vi "Main.vi"(8 "error in":errorcluster, 11 "UART Worker in":refnum<class "UART Worker.lvclass">) -> (0 "error out":errorcluster, 3 "UART Worker out":refnum<class "UART Worker.lvclass">)   [LabVIEW 2020, in "UART Worker.lvclass"]
doc: "The <b>Queued Message Handler</b> of the Worker that owns this VI."
uses:
  UART Worker.lvclass
  C:/Program Files (x86)/National Instruments/LabVIEW 2020/vi.lib/addons/_Workers/Library/Classes/Worker/Worker.lvclass
  rqp_Open Port.ctl
  rqp_Write Buffer.ctl
  Initialization Data.ctl
  Response Cases.ctl
  UART Worker.lvclass/UART Worker.ctl
  rql_readBuffer.ctl
  rql_checkBufferSize.ctl
  rql_checkBufferData.ctl
  rqp_Close Port.ctl
  <vilib>/Utility/error.llb/Error Cluster From Error Code.vi
  <vilib>/ErrorRing/Error Ring.xnode
  <vilib>/addons/_Workers/Library/Classes/Message Queue/Message Queue.lvclass
  3fd13485-57e7-4225-91d7-578f471f1d53.vi
panel:
  in  "stop":bool
  in  "讀取目標字數":i32=1
  in  "Write":bool
  in  "VISA resource name":refnum<visa-resource-name>
  out "read buffer":string
  in  "write buffer":string
  # "1. 設定 VISA\n2. 設定讀取目標字數\n3. 按下”開始通訊”，進行通訊作業\n4. 設定\"write buffer“\n5. 按下\"Write\"，將資料進行寫入\n6. 觀察\"read buffer\"\n7. 按下停止通訊“，結束通訊作業"
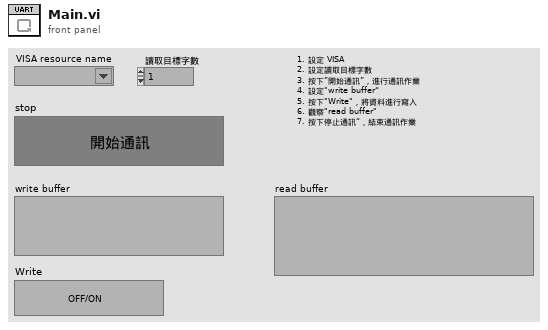
[diagram p1: front panel]
types:
  T1 = typedef "UART Worker.lvclass/Initialization Data.ctl" = cluster{"Response Cases":T2}
  T2 = typedef "UART Worker.lvclass/Response Cases.ctl" = cluster{"Placeholder - Can be deleted":string}
  T3 = typedef "UART Worker.lvclass/rql_checkBufferSize.ctl" = cluster{"Buffer Data":string}
  T4 = typedef "UART Worker.lvclass/rql_readBuffer.ctl" = cluster{"Number of Bytes at Serial Port":u32}
  T5 = typedef "UART Worker.lvclass/rql_checkBufferData.ctl" = cluster{"String":string}
  T6 = typedef "UART Worker.lvclass/rqp_Open Port.ctl" = cluster{"VISA resource name":refnum<visa-resource-name>}
  T7 = typedef "UART Worker.lvclass/rqp_Close Port.ctl" = cluster{"String":string}
  T8 = typedef "UART Worker.lvclass/rqp_Write Buffer.ctl" = cluster{"write buffer":string}
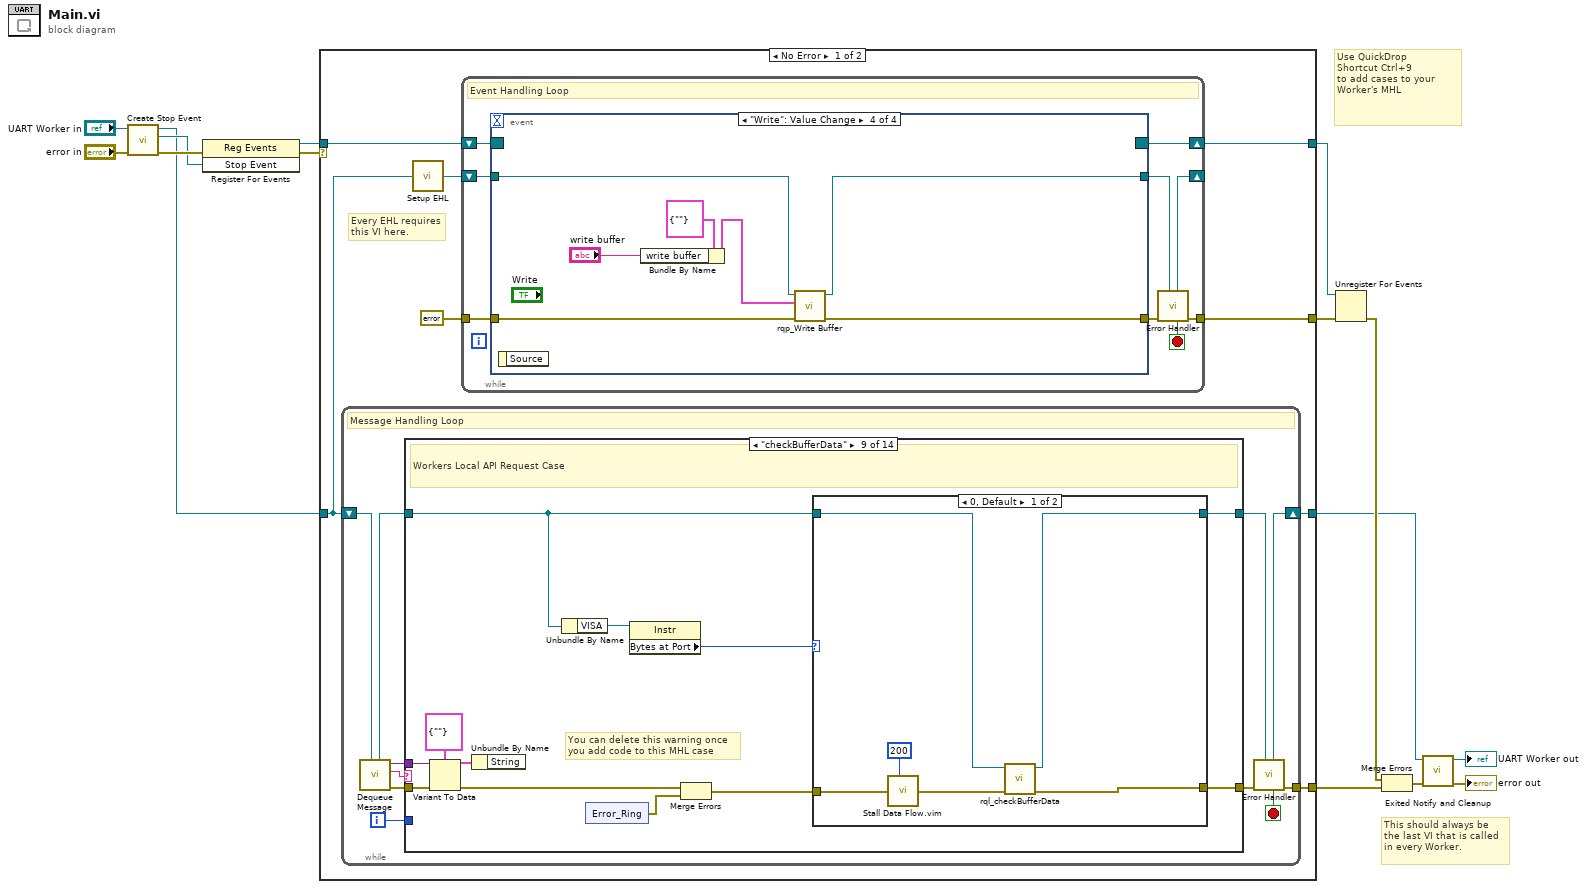
[diagram p0: block diagram]
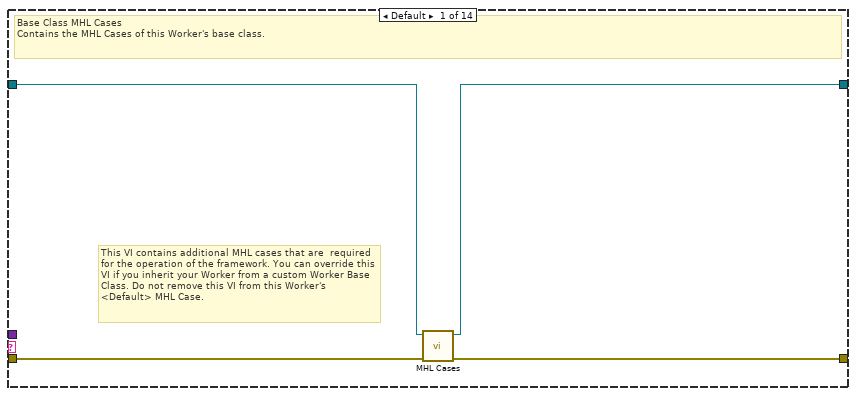
[diagram p2: hidden frame]
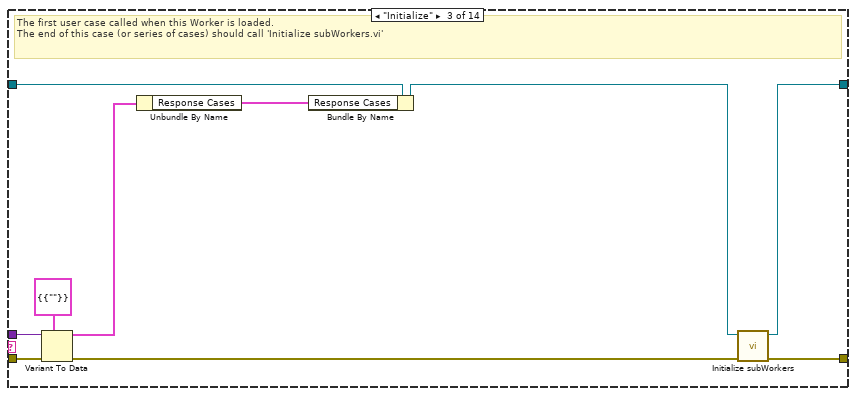
[diagram p4: hidden frame]
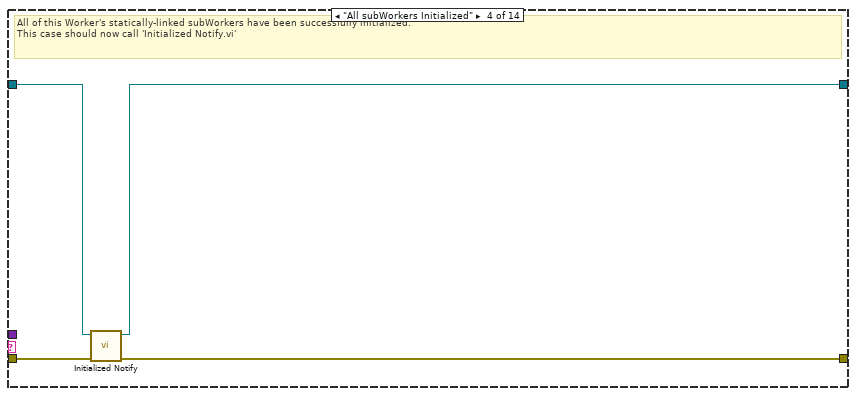
[diagram p5: hidden frame]
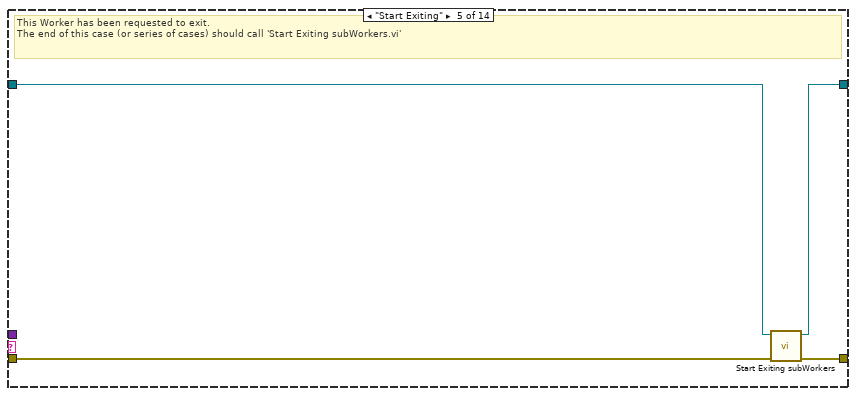
[diagram p6: hidden frame]
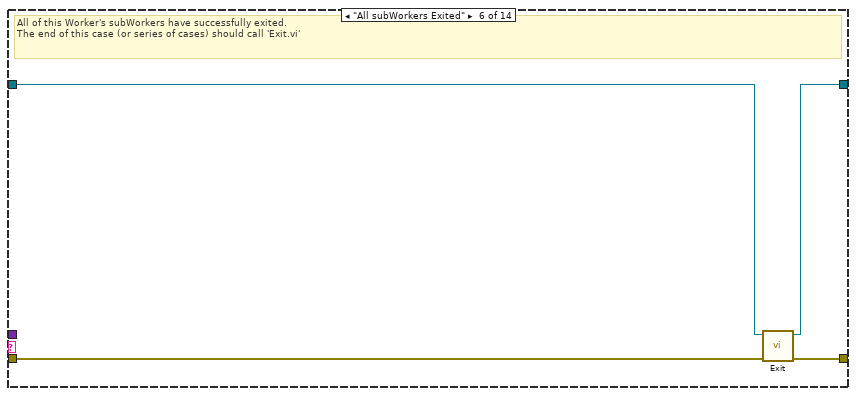
[diagram p7: hidden frame]
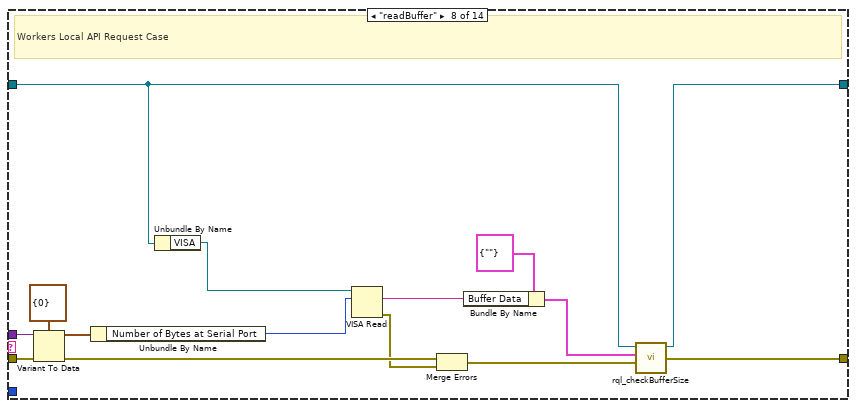
[diagram p9: hidden frame]
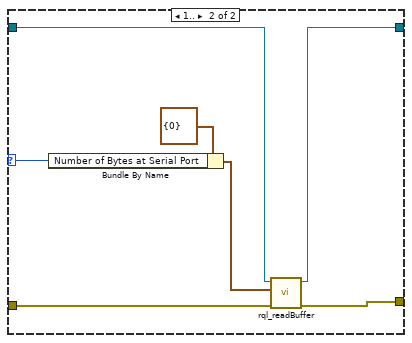
[diagram p10: hidden frame]
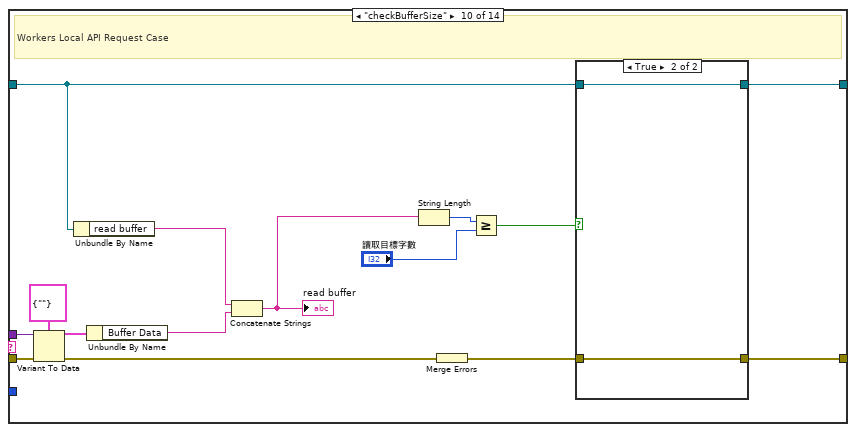
[diagram p11: hidden frame]
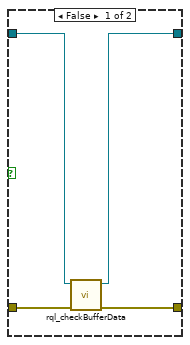
[diagram p12: hidden frame]
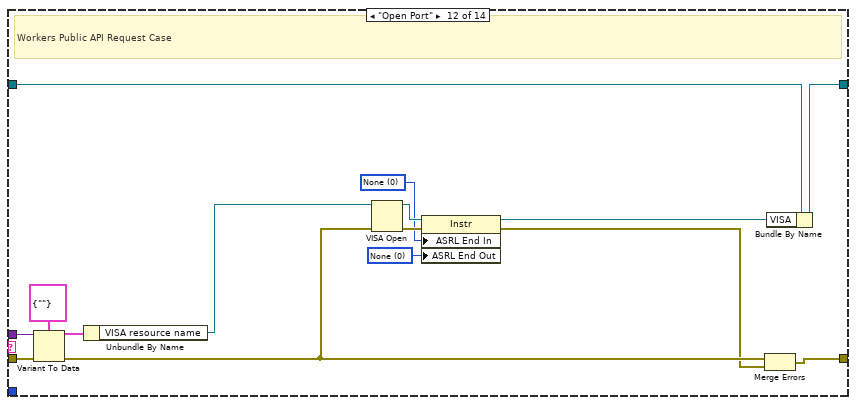
[diagram p14: hidden frame]
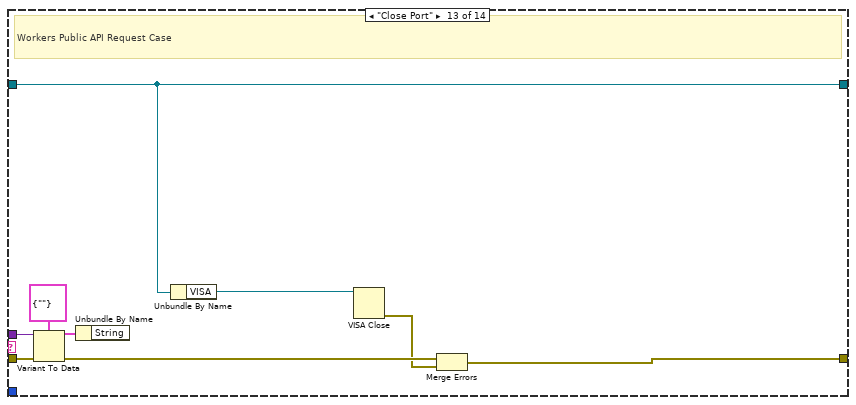
[diagram p15: hidden frame]
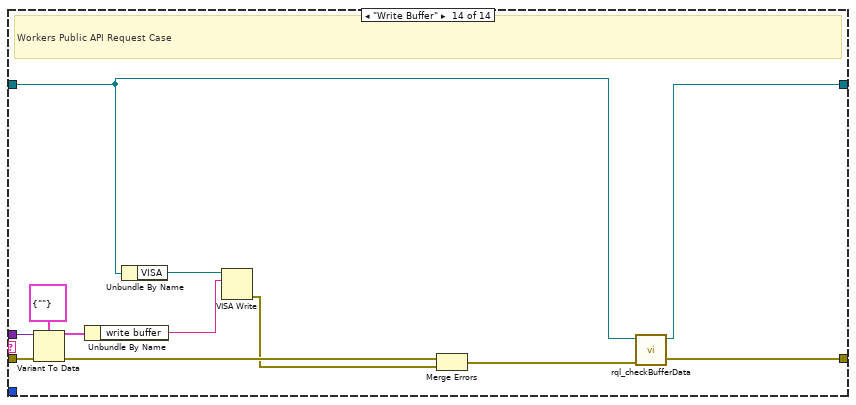
[diagram p16: hidden frame]
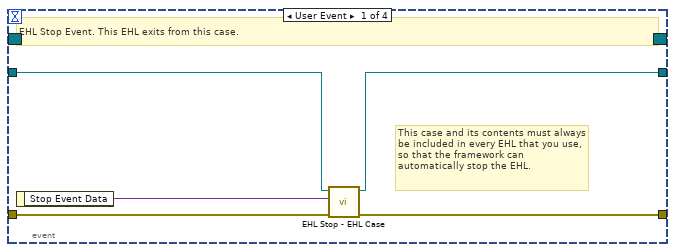
[diagram p17: hidden frame]
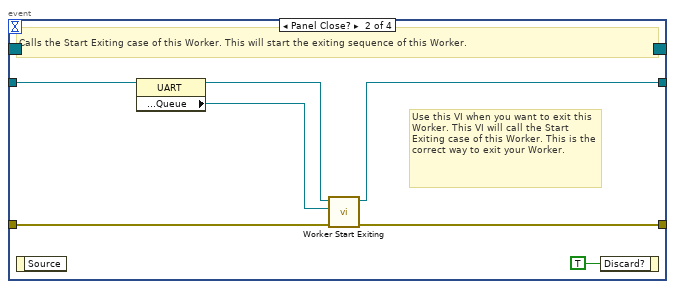
[diagram p18: hidden frame]
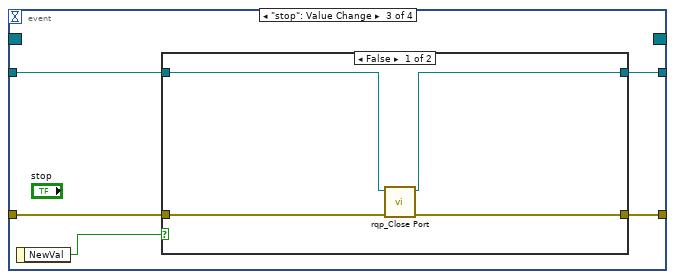
[diagram p19: hidden frame]
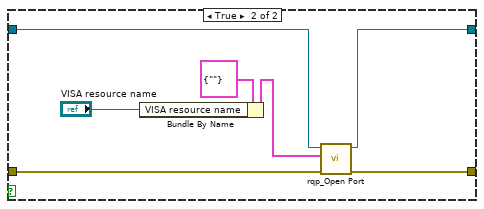
[diagram p20: hidden frame]
diagram:
  # "Use QuickDrop\nShortcut Ctrl+9\nto add cases to your\nWorker's MHL"
  # "This should always be the last VI that is called in every Worker."
  n1 = call-dynamic "Create Stop Event.vi"("error in"="error in", "Worker"="UART Worker in") -> ("error out"=w10:errorcluster, "Stop Event"=w7:refnum<user-event>, "Worker out"=w4:refnum<class "UART Worker.lvclass">)  [unwired: 7 in]
  n2 = register-events(error in=w10, w7) -> (reference out=w9:refnum<event-registration>, error out=w1:errorcluster)  [unwired: 1 in]
  n3 = case shown="No Error" w1 {
    tunnel: w4 -> [w18 w214]
    tunnel: [w16 w215] -> w8
    tunnel: w9 -> [w23 w216]
    tunnel: [w20 w217] -> w14
    tunnel: [w22 w216] -> w13
    tunnel: [w17 w213] -> w11
    selector: w1 -> [_ w217]
    frame No Error {
      # "Every EHL requires\nthis VI here."
      n4 = while {
        shift-right: [w32] -> w17
        shift-left: w18 -> [w34]
        tunnel: [w33] -> w16
        i -> [w25]
        stop <- w26 stop-if-true
        # "Message Handling Loop"
        n5 = call-dynamic "Dequeue Message.vi"("Worker"=w34) -> ("error out"=w31:errorcluster, "Case out"=w27:string, "Data out"=w24:variant, "Worker out"=w29:refnum<class "UART Worker.lvclass">)  [unwired: 6 in, 1 out]
        n6 = case "Worker MHL Case Structure (DO NOT CHANGE LABEL NAME)" shown="\"checkBufferData\"" w27 {
          tunnel: w31 -> [w38 w39 w48 w52 w55 w62 w64 w79 w91 w124 w132 w146 w156 w168]
          tunnel: [w37 w39 w50 w51 w58 w61 w64 w70 w81 w113 w132 w142 w151 w159] -> w30
          tunnel: w29 -> [w36 w40 w47 w54 w56 w60 w63 w68 w83 w111 w131 w147 w149 w157]
          tunnel: [w35 w40 w49 w53 w57 w59 w63 w69 w84 w112 w131 w134 w149 w158] -> w28
          tunnel: w25 -> [_ _ _ _ _ _ _ _ _ _ _ _ _ _]
          tunnel: w24 -> [_ _ w45 _ _ _ _ w76 w88 w121 _ w144 w153 w165]
          frame Default {
            # "This VI contains additional MHL cases that are  required for the operation of the framework. You can override this VI if you inherit your Worker from a custom Worker Base Class. Do not remove this VI from this Worker's <Default> MHL Case."
            # "Base Class MHL Cases\nContains the MHL Cases of this Worker's base class."
            n7 = call-dynamic "MHL Cases.vi"("error in"=w38, "Worker in"=w36) -> ("error out"=w37:errorcluster, "Worker out"=w35:refnum<class "UART Worker.lvclass">)  [unwired: 8 in]
          }
          frame "------------ FRAMEWORK CASES -----------" {
            # "Start of Workers Framework Cases"
          }
          frame "Initialize" {
            # "The first user case called when this Worker is loaded.\nThe end of this case (or series of cases) should call 'Initialize subWorkers.vi'"
            n8 = Variant To Data(error in=w48, type=T1 {"Response Cases"={"Placeholder - Can be deleted"=""}} ("Initialization Data"), Variant=w45) -> (data=w43:T1, error out=w46:errorcluster)
            n9 = Unbundle By Name(w43) -> ("Response Cases"=w42:T2)
            n10 = Bundle By Name(cluster=w47, "Response Cases"=w42) -> (w44:refnum<class "UART Worker.lvclass">)
            n11 = call-dynamic "Initialize subWorkers.vi"("error in"=w46, "Worker"=w44) -> ("error out"=w50:errorcluster, "dup Worker out"=w49:refnum<class "UART Worker.lvclass">)  [unwired: 8 in]
          }
          frame "All subWorkers Initialized" {
            # "All of this Worker's statically-linked subWorkers have been successfully initialized.\nThis case should now call 'Initialized Notify.vi'"
            n12 = call-dynamic "Initialized Notify.vi"("error in"=w52, "Worker"=w54) -> ("error out"=w51:errorcluster, "dup Worker out"=w53:refnum<class "UART Worker.lvclass">)  [unwired: 8 in]
          }
          frame "Start Exiting" {
            # "This Worker has been requested to exit. \nThe end of this case (or series of cases) should call 'Start Exiting subWorkers.vi'"
            n13 = call-dynamic "Start Exiting subWorkers.vi"("error_in"=w55, "Worker"=w56) -> ("error out"=w58:errorcluster, "dup Worker out"=w57:refnum<class "UART Worker.lvclass">)  [unwired: 8 in]
          }
          frame "All subWorkers Exited" {
            # "All of this Worker's subWorkers have successfully exited. \nThe end of this case (or series of cases) should call 'Exit.vi'"
            n14 = call-dynamic "Exit.vi"("error_in"=w62, "Worker"=w60) -> ("error out"=w61:errorcluster, "dup Worker out"=w59:refnum<class "UART Worker.lvclass">)  [unwired: 8 in]
          }
          frame "------------- LOCAL API CASES -------------" {
            # "Start of Workers Local API Cases"
          }
          frame "readBuffer" {
            # "Workers Local API Request Case"
            n15 = Variant To Data(error in=w79, type=T4 {"Number of Bytes at Serial Port"=0} ("Data"), Variant=w76) -> (data=w74:T4, error out=w78:errorcluster)
            n16 = Unbundle By Name(w74) -> ("Number of Bytes at Serial Port"=w71:u32)
            n17 = Unbundle By Name(w68) -> ("VISA"=w72:refnum<visa-resource-name>)
            n18 = VISA Read(VISA resource name=w72, byte count=w71) -> (read buffer=w65:string, error out=w73:errorcluster)  [unwired: 1 in, 2 out]
            n19 = Merge Errors(w78, w73) -> (w75:errorcluster)
            n20 = Bundle By Name(cluster=T3 {"Buffer Data"=""} ("Data in"), "Buffer Data"=w65) -> (w66:T3)
            n21 = call "rql_checkBufferSize.vi"("error in"=w75, "Data in"=w66, "UART Worker in"=w68) -> ("error out"=w70:errorcluster, "dup UART Worker out"=w69:refnum<class "UART Worker.lvclass">)  [unwired: 7 in]
          }
          frame "checkBufferData" {
            # "You can delete this warning once\nyou add code to this MHL case"
            # "Workers Local API Request Case"
            n22 = Variant To Data(error in=w91, type=T5 {"String"=""} ("Data"), Variant=w88) -> (data=w87:T5, error out=w90:errorcluster)
            n23 = Unbundle By Name(w87) -> ()  [unwired: 1 out]
            n24 = Unbundle By Name(w83) -> ("VISA"=w85:refnum<visa-resource-name>)
            n25 = xnode ("Error_Ring")() -> ("error out"=w86:errorcluster)
            n26 = property class="Instr"(reference=w85) -> ("Bytes at Port"=w80:u32)  [unwired: 1 in, 2 out]
            n27 = Merge Errors(w90, w86) -> (w82:errorcluster)
            n28 = case shown="0, Default" w80 {
              selector: w80 -> [_ w98]
              tunnel: [w97 w104] -> w84
              tunnel: w83 -> [w96 w103]
              tunnel: w82 -> [w94 w102]
              tunnel: [w95 w101] -> w81
              frame 0, Default {
                n29 = call "Stall Data Flow.vim"("value in"=w94, "milliseconds to wait"=u32 200) -> ("value out"=w93:errorcluster)  [unwired: 1 out]
                n30 = call "rql_checkBufferData.vi"("error in"=w93, "UART Worker in"=w96) -> ("error out"=w95:errorcluster, "dup UART Worker out"=w97:refnum<class "UART Worker.lvclass">)  [unwired: 8 in]
              }
              frame 1.. {
                n31 = Bundle By Name(cluster=T4 {"Number of Bytes at Serial Port"=0} ("Data in"), "Number of Bytes at Serial Port"=w98) -> (w99:T4)
                n32 = call "rql_readBuffer.vi"("error in"=w102, "Data in"=w99, "UART Worker in"=w103) -> ("error out"=w101:errorcluster, "dup UART Worker out"=w104:refnum<class "UART Worker.lvclass">)  [unwired: 7 in]
              }
            }
          }
          frame "checkBufferSize" {
            # "Workers Local API Request Case"
            n33 = Variant To Data(error in=w124, type=T3 {"Buffer Data"=""} ("Data"), Variant=w121) -> (data=w120:T3, error out=w123:errorcluster)
            n34 = Unbundle By Name(w111) -> ("read buffer"=w117:string)
            n35 = Unbundle By Name(w120) -> ("Buffer Data"=w118:string)
            n36 = Concatenate Strings(w117, w118) -> (w116:string)
            "read buffer" <- w116
            n37 = String Length(string=w116) -> (length=w115:i32)
            n38 = Merge Errors(w123) -> (w119:errorcluster)
            n39 = Greater Or Equal?(x=w115, y="讀取目標字數") -> (x >= y?=w110:bool)
            n40 = case shown="True" w110 {
              tunnel: w119 -> [w128 w129]
              tunnel: [w127 w129] -> w113
              tunnel: [w126 w130] -> w112
              tunnel: w111 -> [w125 w130]
              frame False {
                n41 = call "rql_checkBufferData.vi"("error in"=w128, "UART Worker in"=w125) -> ("error out"=w127:errorcluster, "dup UART Worker out"=w126:refnum<class "UART Worker.lvclass">)  [unwired: 8 in]
              }
              frame True {
              }
            }
          }
          frame "------------- PUBLIC API CASES -------------" {
            # "Start of Workers Public API Cases"
          }
          frame "Open Port" {
            w138 = u16 0 items=["None", "Last Bit", "TermChar", "Break"] ("Serial Settings:End Mode for Writes")
            w139 = u16 0 items=["None", "Last Bit", "TermChar"] ("Serial Settings:End Mode for Reads")
            # "Workers Public API Request Case"
            n42 = Variant To Data(error in=w146, type=T6 {"VISA resource name"=""} ("Data"), Variant=w144) -> (data=w143:T6, error out=w136:errorcluster)
            n43 = Unbundle By Name(w143) -> ("VISA resource name"=w137:refnum<visa-resource-name>)
            n44 = VISA Open(error in (no error)=w136, VISA resource name=w137) -> (VISA resource name=w141:refnum<visa-resource-name>, error out=w140:errorcluster)  [unwired: 3 in]
            n45 = property class="Instr"(reference=w141, error in=w140, "ASRL End In"=w139, "ASRL End Out"=w138) -> (reference out=w133:refnum<visa-resource-name>, error out=w135:errorcluster)
            n46 = Merge Errors(w136, w135) -> (w142:errorcluster)
            n47 = Bundle By Name(cluster=w147, "VISA"=w133) -> (w134:refnum<class "UART Worker.lvclass">)
          }
          frame "Close Port" {
            # "Workers Public API Request Case"
            n48 = Variant To Data(error in=w156, type=T7 {"String"=""} ("Data"), Variant=w153) -> (data=w152:T7, error out=w155:errorcluster)
            n49 = Unbundle By Name(w152) -> ()  [unwired: 1 out]
            n50 = Unbundle By Name(w149) -> ("VISA"=w148:refnum<visa-resource-name>)
            n51 = VISA Close(VISA resource name=w148) -> (error out=w150:errorcluster)  [unwired: 1 in]
            n52 = Merge Errors(w155, w150) -> (w151:errorcluster)
          }
          frame "Write Buffer" {
            # "Workers Public API Request Case"
            n53 = Variant To Data(error in=w168, type=T8 {"write buffer"=""} ("Data"), Variant=w165) -> (data=w164:T8, error out=w167:errorcluster)
            n54 = Unbundle By Name(w164) -> ("write buffer"=w162:string)
            n55 = Unbundle By Name(w157) -> ("VISA"=w161:refnum<visa-resource-name>)
            n56 = VISA Write(VISA resource name=w161, write buffer=w162) -> (error out=w160:errorcluster)  [unwired: 1 in, 2 out]
            n57 = Merge Errors(w167, w160) -> (w163:errorcluster)
            n58 = call "rql_checkBufferData.vi"("error in"=w163, "UART Worker in"=w157) -> ("error out"=w159:errorcluster, "dup UART Worker out"=w158:refnum<class "UART Worker.lvclass">)  [unwired: 8 in]
          }
        }
        n59 = call-dynamic "Error Handler.vi"("Worker"=w28, "error_in"=w30) -> ("error out"=w33:errorcluster, "Stop Loop"=w26:bool, "Worker out"=w32:refnum<class "UART Worker.lvclass">)  [unwired: 7 in]
      }
      n60 = call-dynamic "Setup EHL.vi"("Worker"=w18) -> ("Worker out"=w19:refnum<class "UART Worker.lvclass">)  [unwired: 14 in]
      n61 = while "Event Handling Loop" {
        shift-right: [w177] -> w22
        shift-left: w23 -> [w176]
        tunnel: [w172] -> w20
        tunnel: errorcluster {"status"=FALSE, "code"=0, "source"=""} ("error constant") -> [w174]
        shift-right: [w170] -> _
        shift-left: w19 -> [w175]
        stop <- w169 stop-if-true
        # "Event Handling Loop"
        n62 = event shown="[3] \"Write\": Value Change" {
          selector: w176 -> [_ _ _ _]
          dyn-events: [_ _ _ _] -> w177
          timeout: _ -> [_ _ _ _]
          tunnel: [w181 w188 w193 w210] -> w173
          tunnel: w174 -> [w182 w187 w194 w209]
          tunnel: w175 -> [w180 w186 w192 w211]
          tunnel: [w179 w185 w191 w212] -> w171
          event User Event {
            # "This case and its contents must always be included in every EHL that you use, so that the framework can automatically stop the EHL."
            # "EHL Stop Event. This EHL exits from this case."
            n63 = event-data() -> ("Stop Event Data"=w178:variant)  [unwired: 1 in]
            n64 = call-dynamic "EHL Stop - EHL Case.vi"("error in"=w182, "Stop Event Data"=w178, "Worker"=w180) -> ("error out"=w181:errorcluster, "Worker out"=w179:refnum<class "UART Worker.lvclass">)  [unwired: 7 in]
          }
          event Panel Close? {
            # "Use this VI when you want to exit this Worker. This VI will call the Start Exiting case of this Worker. This is the correct way to exit your Worker."
            # "Calls the Start Exiting case of this Worker. This will start the exiting sequence of this Worker."
            n65 = event-data() -> ()  [unwired: 1 in, 1 out]
            n66 = property class="UART"(reference=w186) -> (reference out=w184:refnum<class "UART Worker.lvclass">, "Accessors:Read:Public API:Queue"=w183:refnum<class "Message Queue.lvclass">)  [unwired: 1 in, 1 out]
            n67 = call-dynamic "Worker Start Exiting.vi"("error_in"=w187, "Message Queue"=w183, "Worker"=w184) -> ("error out"=w188:errorcluster, "dup Worker out"=w185:refnum<class "UART Worker.lvclass">)  [unwired: 7 in]
            n68 = event-data("Discard?"=TRUE) -> ()  [unwired: 1 in, 1 out]
          }
          event "stop": Value Change {
            n69 = event-data() -> ("NewVal"=w190:bool)  [unwired: 1 in]
            n70 = case shown="False" w190 {
              tunnel: w194 -> [w196 w205]
              tunnel: [w195 w204] -> w193
              tunnel: w192 -> [w198 w203]
              tunnel: [w197 w202] -> w191
              frame False {
                n71 = call "rqp_Close Port.vi"("error in"=w196, "UART Worker in"=w198) -> ("error out"=w195:errorcluster, "dup UART Worker out"=w197:refnum<class "UART Worker.lvclass">)  [unwired: 7 in, 1 out]
              }
              frame True {
                n72 = Bundle By Name(cluster=T6 {"VISA resource name"=""} ("Data in"), "VISA resource name"="VISA resource name") -> (w200:T6)
                n73 = call "rqp_Open Port.vi"("error in"=w205, "Data in"=w200, "UART Worker in"=w203) -> ("error out"=w204:errorcluster, "dup UART Worker out"=w202:refnum<class "UART Worker.lvclass">)  [unwired: 6 in, 1 out]
              }
            }
          }
          event "Write": Value Change {
            n74 = event-data() -> ()  [unwired: 1 in, 1 out]
            n75 = Bundle By Name(cluster=T8 {"write buffer"=""} ("Data in"), "write buffer"="write buffer") -> (w207:T8)
            n76 = call "rqp_Write Buffer.vi"("error in"=w209, "Data in"=w207, "UART Worker in"=w211) -> ("error out"=w210:errorcluster, "dup UART Worker out"=w212:refnum<class "UART Worker.lvclass">)  [unwired: 6 in, 1 out]
          }
        }
        n77 = call-dynamic "Error Handler.vi"("Worker"=w171, "error_in"=w173) -> ("error out"=w172:errorcluster, "Stop Loop"=w169:bool, "Worker out"=w170:refnum<class "UART Worker.lvclass">)  [unwired: 7 in]
      }
    }
    frame Error {
      n78 = call-dynamic "Error Handler.vi"("Worker"=w214, "error_in"=w217) -> ("error out"=w215:errorcluster, "Worker out"=w213:refnum<class "UART Worker.lvclass">)  [unwired: 7 in, 1 out]
    }
  }
  n79 = Unregister For Events(event registration refnum=w13, error in=w14) -> (error out=w15:errorcluster)
  n80 = Merge Errors(w15, w8) -> (w12:errorcluster)
  n81 = call-dynamic "Exited Notify and Cleanup.vi"("error_in"=w12, "Worker"=w11) -> ("error out"=→"error out":errorcluster, "dup Worker out"=→"UART Worker out":refnum<class "UART Worker.lvclass">)  [unwired: 8 in]
